vi "SVN_GetLog.vi"(5 "rev End":i32=-2, 7 "rev Start":i32, 8 "Error In":errorcluster, 11 "repo path":path=path "") -> (0 "Error Out":errorcluster, 3 "SVN Log-Info_Cluster[]":T1[](array[typedef]))   [LabVIEW 2014]
uses:
  controls/SVN_LogEntry_Cluster.ctl
panel:
  out "cmd command":string
  out "standard output":string
  out "standard error":string
  # "DATE -1\nHEAD -2\nBASE -3\nCOMMITED -4\nPREV -5"
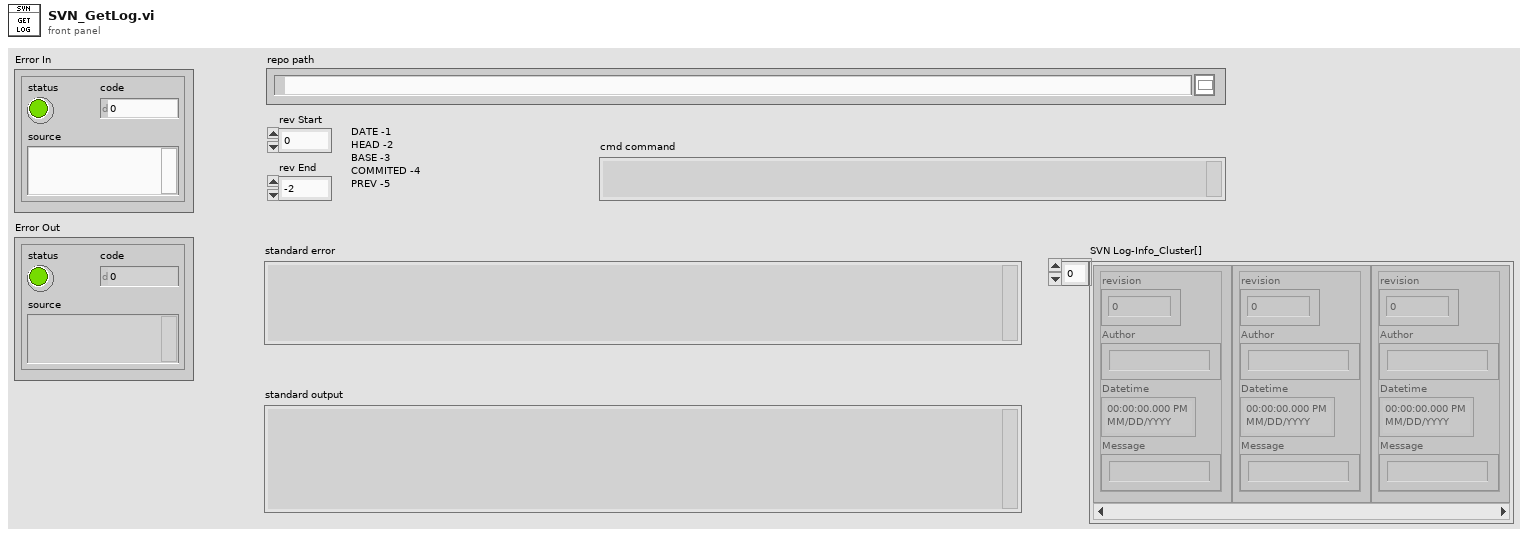
[diagram p1: front panel]
types:
  T1 = typedef "SVN_LogEntry_Cluster.ctl" = cluster{"revision":i32, "Author":string, "Datetime":timestamp, "Message":string}
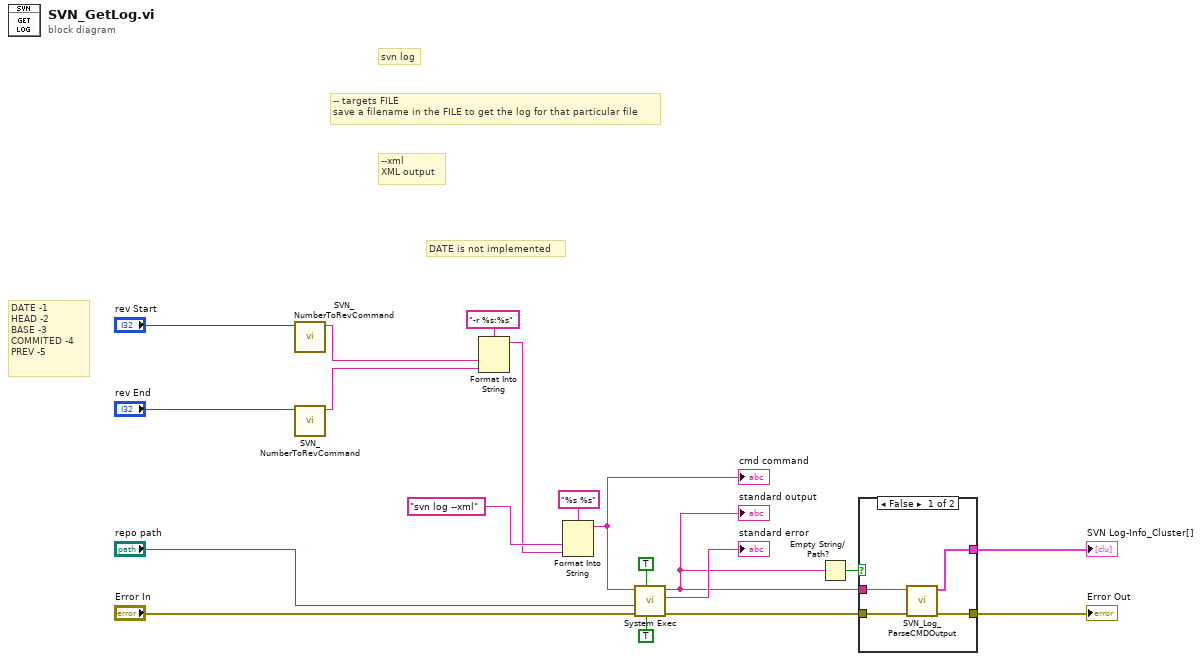
[diagram p0: block diagram]
diagram:
  # "DATE is not implemented"
  # "DATE -1\nHEAD -2\nBASE -3\nCOMMITED -4\nPREV -5"
  # "--xml\nXML output"
  # "-- targets FILE \nsave a filename in the FILE to get the log for that particular file"
  # "svn log"
  n1 = call "SVN_NumberToRevCommand.vi"("rev End"="rev Start") -> ("String"=w3:string)  [unwired: 10 in]
  n2 = call "SVN_NumberToRevCommand.vi"("rev End"="rev End") -> ("String"=w2:string)  [unwired: 10 in]
  n3 = Format Into String(format string="-r %s:%s", w3, w2) -> (resulting string=w11:string)  [unwired: 2 in, 1 out]
  n4 = Format Into String(format string="%s %s", "svn log --xml" ("command line"), w11) -> (resulting string=w9:string)  [unwired: 2 in, 1 out]
  "cmd command" <- w9
  n5 = call <vilib>:"System Exec.vi"("run minimized? (F)"=TRUE, "wait until completion? (T)"=TRUE, "error in (no error)"="Error In", "working directory"="repo path", "command line"=w9) -> ("error out"=w7:errorcluster, "standard error"=→"standard error":string, "standard output"=w10:string)  [unwired: 3 in, 1 out]
  "standard output" <- w10
  n6 = Empty String/Path?(string/path=w10) -> (empty?=w8:bool)
  n7 = case shown="False" w8 {
    tunnel: w10 -> [w23 _]
    tunnel: w7 -> [w22 w24]
    tunnel: [w21 w24] -> w6
    tunnel: [w20 _] -> w5
    frame False {
      n8 = call "SVN_Log_ParseCMDOutput.vi"("Error In"=w22, "SVN_Log_XML (In)"=w23) -> ("Error Out"=w21:errorcluster, "SVN Log-Info_Cluster[]"=w20:T1[])  [unwired: 8 in]
    }
    frame True {
    }
  }
  "Error Out" <- w6
  "SVN Log-Info_Cluster[]" <- w5
